vi "Periodic Tasks.vi"(11 "error in (no error)":errorcluster) -> ()   [LabVIEW 2012]
doc: "This VI runs in parallel to other tasks. It can contain as many user-defined periodic loops as you need. These can carry out PID or other sorts of timed response."
uses:
  <vilib>/Rock Robotics/WPI/DriverStation/DriverStationLCD/WPI_DriverStationLCDLCDLine.ctl
  <vilib>/Rock Robotics/SystemInterfaces/Utilities/FPGA_UtilitiesLED Source.ctl
  <vilib>/Rock Robotics/SystemInterfaces/Utilities/FPGA_UtilitiesLED State.ctl
  Robot Global Data.vi
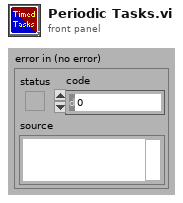
[diagram p1: front panel]
types:
  T1 = typedef "FPGA_UtilitiesLED State.ctl" = enum16{"Off", "On", "Toggle"}
  T2 = typedef "FPGA_UtilitiesLED Source.ctl" = enum16{"User LED", "FPGA LED"}
  T3 = typedef "WPI_DriverStationLCDLCDLine.ctl" = enum16{"Main - Line 1", "User - Line 2", "User - Line 3", "User - Line 4", "User - Line 5", "User - Line 6"}
  T4 = cluster{"Case":dbl, "VisionTrack":bool, "ShootEnableWheels":bool, "Shoot":bool, "ManualExtend":dbl, "ManualRotate":dbl, "YCoord":dbl, "FlipUp":bool, "RotDeadband":dbl, "ExtDeadband":dbl, "ExtPOT":dbl, "RotPOT":dbl, "WheelFSpd":dbl, "WheelBSpd":dbl, "ServoPositions":cluster{"FlipperLeftUp":dbl, "FlipperLeftDown":dbl, "FlipperRightUp":dbl, "FlipperRightDown":dbl, "KickerLeftBack":dbl, "KickerLeftForward":dbl, "KickerRightBack":dbl, "KickerRightForward":dbl}, "POTPositions":cluster{"Setpoint 1":dbl, "Setpoint 2":dbl, "Setpoint 3":dbl, "Setpoint 4":dbl, "RotLow":dbl, "RotHigh":dbl, "ExtLow":dbl, "ExtHigh":dbl}, "ClimberHooked":bool}
  T5 = typedef "WPI_DigitalInputDevRef.ctl" = cluster{"DevStatus":errorcluster, "DIO Channel":T6, "Digital Module":T7}
  T6 = typedef "FPGA_DIOChannel.ctl" = enum8{"DIO 1", "DIO 2", "DIO 3", "DIO 4", "DIO 5", "DIO 6", "DIO 7", "DIO 8", "DIO 9", "DIO 10", "DIO 11", "DIO 12", "DIO 13", "DIO 14", "Invalid"}
  T7 = typedef "FPGA_TypedefDigitalModule.ctl" = enum16{"Digital Module 1", "Digital Module 2"}
  T8 = typedef "WPI_AnalogChannelDevRef.ctl" = cluster{"DevStatus":errorcluster, "Analog Module":T9, "Analog Channel":T10}
  T9 = typedef "FPGA_TypedefAnalogModule.ctl" = enum16{"Analog Module 1", "Analog Module 2"}
  T10 = typedef "FPGA_AIChannel.ctl" = enum8{"AI 1", "AI 2", "AI 3", "AI 4", "AI 5", "AI 6", "AI 7", "AI 8", "Invalid"}
  T11 = cluster{"FlipperLeftUp":dbl, "FlipperLeftDown":dbl, "FlipperRightUp":dbl, "FlipperRightDown":dbl, "KickerLeftBack":dbl, "KickerLeftForward":dbl, "KickerRightBack":dbl, "KickerRightForward":dbl}
  T12 = cluster{"Setpoint 1":dbl, "Setpoint 2":dbl, "Setpoint 3":dbl, "Setpoint 4":dbl, "RotLow":dbl, "RotHigh":dbl, "ExtLow":dbl, "ExtHigh":dbl}
  T13 = typedef "WPI_RelayValue.ctl" = enum16{"Off", "On", "Forward", "Reverse"}
  T14 = cluster{"Case":dbl, "Extension":dbl, "Rotation":dbl, "WheelF":dbl, "WheelB":dbl, "Left Kicker":dbl, "Right Kicker":dbl, "Left Flipper":dbl, "Right Flipper":dbl, "Lights":T13}
  T15 = typedef "WPI_GyroDevRef.ctl" = cluster{"DevStatus":errorcluster, "Analog Module":T9, "Analog Channel":T10, "Offset":dbl, "Gain (VoltsPerDegree/Second)":dbl}
  T16 = typedef "WPI_EncoderDevRef.ctl" = cluster{"DevStatus":errorcluster, "EncoderIndex":T17, "CounterIndex":T18, "DistancePerCount":dbl, "Decoding Type":T19}
  T17 = typedef "FPGA_EncoderIdx.ctl" = enum8{"Enc 0", "Enc 1", "Enc 2", "Enc 3", "Invalid"}
  T18 = typedef "FPGA_CounterCtrSystemIndex.ctl" = enum8{"Ctr 0", "Ctr 1", "Ctr 2", "Ctr 3", "Ctr 4", "Ctr 5", "Ctr 6", "Ctr 7", "Invalid"}
  T19 = typedef "WPI_EncoderType.ctl" = enum16{"1x", "2x", "4x"}
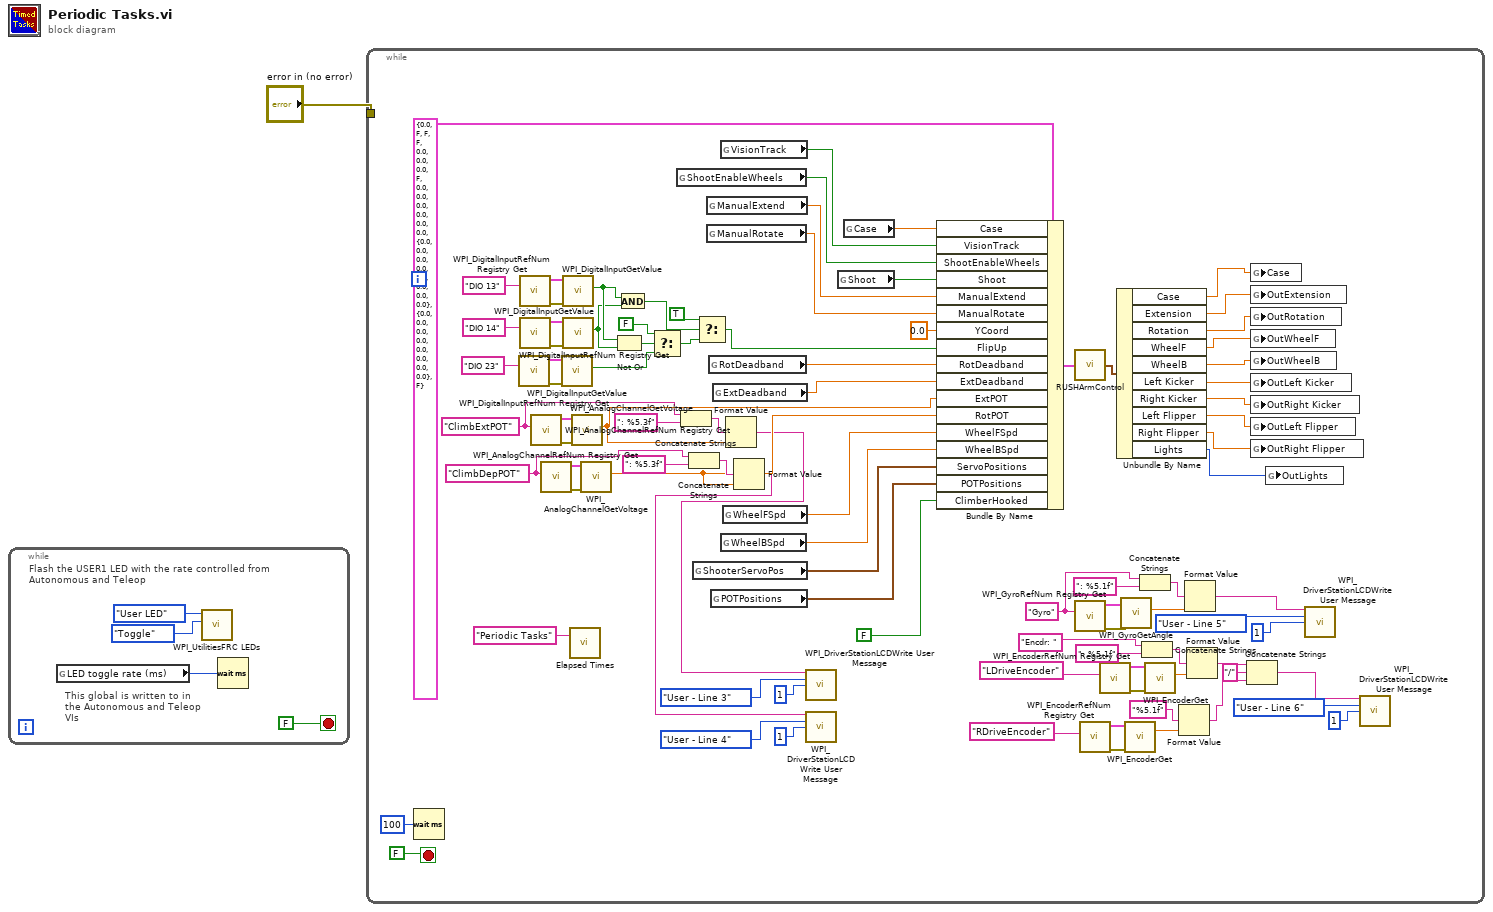
[diagram p0: block diagram]
diagram:
  n1 = while {
    stop <- FALSE stop-if-true
    # "This global is written to in the Autonomous and Teleop VIs"
    # "Flash the USER1 LED with the rate controlled from Autonomous and Teleop"
    n2 = global read "Robot Global Data.vi" "LED toggle rate (ms)"() -> (w2:u32)
    n3 = call <vilib>:"WPI_UtilitiesFRC LEDs.vi"("State"=FPGA_UtilitiesLED_State."Toggle", "LED Type"=FPGA_UtilitiesLED_Source."User LED") -> ()  [unwired: 1 in, 9 out]
    n4 = Wait (ms)(milliseconds to wait=w2) -> ()  [unwired: 1 out]
  }
  n5 = while {
    tunnel: "error in (no error)" -> [_]
    stop <- FALSE stop-if-true
    w55 = "ClimbExtPOT" ("refnum name")
    w51 = "ClimbDepPOT" ("refnum name")
    w41 = "Gyro" ("refnum name")
    n6 = Wait (ms)(milliseconds to wait=u32 100) -> ()  [unwired: 1 out]
    n7 = call <vilib>:"WPI_DigitalInputRefNum Registry Get.vi"("refnum name"="DIO 23") -> ("error out"=w24:errorcluster, "DigitalInputDevRef"=w22:T5)  [unwired: 9 in]
    n8 = call <vilib>:"WPI_DigitalInputRefNum Registry Get.vi"("refnum name"="DIO 13") -> ("error out"=w20:errorcluster, "DigitalInputDevRef"=w19:T5)  [unwired: 9 in]
    n9 = call <vilib>:"WPI_DigitalInputRefNum Registry Get.vi"("refnum name"="DIO 14") -> ("error out"=w15:errorcluster, "DigitalInputDevRef"=w16:T5)  [unwired: 9 in]
    n10 = call <vilib>:"WPI_AnalogChannelRefNum Registry Get.vi"("refnum name"=w55) -> ("error out"=w27:errorcluster, "AIDeviceRef"=w21:T8)  [unwired: 9 in]
    n11 = call <vilib>:"WPI_AnalogChannelRefNum Registry Get.vi"("refnum name"=w51) -> ("error out"=w26:errorcluster, "AIDeviceRef"=w25:T8)  [unwired: 9 in]
    n12 = call <vilib>:"WPI_DigitalInputGetValue.vi"("error in (no error)"=w24, "DigitalInputDevRef"=w22) -> ("Value"=w64:bool)  [unwired: 7 in, 2 out]
    n13 = call <vilib>:"WPI_DigitalInputGetValue.vi"("error in (no error)"=w20, "DigitalInputDevRef"=w19) -> ("Value"=w14:bool)  [unwired: 7 in, 2 out]
    n14 = call <vilib>:"WPI_DigitalInputGetValue.vi"("error in (no error)"=w15, "DigitalInputDevRef"=w16) -> ("Value"=w13:bool)  [unwired: 7 in, 2 out]
    n15 = call "Elapsed Times.vi"("Call Name"="Periodic Tasks") -> ()  [unwired: 2 in, 1 out]
    n16 = call <vilib>:"WPI_AnalogChannelGetVoltage.vi"("error in (no error)"=w27, "AIDeviceRef"=w21) -> ("Voltage"=w56:dbl)  [unwired: 7 in, 2 out]
    n17 = call <vilib>:"WPI_AnalogChannelGetVoltage.vi"("error in (no error)"=w26, "AIDeviceRef"=w25) -> ("Voltage"=w52:dbl)  [unwired: 7 in, 2 out]
    n18 = Not Or(1:w13, 2:w14) -> (0:w68:bool)
    n19 = And(x=w14, y=w13) -> (x .and. y?=w70:bool)
    n20 = Select(t=FALSE, s=w68, f=w64) -> (s? t:f=w66:bool)
    n21 = global read "Robot Global Data.vi" "ShootEnableWheels"() -> (w90:bool)
    n22 = Concatenate Strings(w55, ": %5.3f") -> (w57:string)
    n23 = Concatenate Strings(w51, ": %5.3f") -> (w54:string)
    n24 = global read "Robot Global Data.vi" "ShooterServoPos"() -> (w82:T11)
    n25 = Select(t=TRUE, s=w70, f=w66) -> (s? t:f=w65:bool)
    n26 = global read "Robot Global Data.vi" "ManualExtend"() -> (w88:dbl)
    n27 = global read "Robot Global Data.vi" "ManualRotate"() -> (w87:dbl)
    n28 = global read "Robot Global Data.vi" "RotDeadband"() -> (w86:dbl)
    n29 = global read "Robot Global Data.vi" "POTPositions"() -> (w81:T12)
    n30 = global read "Robot Global Data.vi" "ExtDeadband"() -> (w85:dbl)
    n31 = global read "Robot Global Data.vi" "VisionTrack"() -> (w91:bool)
    n32 = global read "Robot Global Data.vi" "WheelBSpd"() -> (w83:dbl)
    n33 = global read "Robot Global Data.vi" "WheelFSpd"() -> (w84:dbl)
    n34 = Format Value(format string=w57, value (0)=w56) -> (output string=w50:string)  [unwired: 1 in]
    n35 = Format Value(format string=w54, value (0)=w52) -> (output string=w49:string)  [unwired: 1 in]
    n36 = call <vilib>:"WPI_DriverStationLCDWrite User Message.vi"("line text"=w50, "line"=WPI_DriverStationLCDLCDLine."User - Line 3", "starting column"=i8 1) -> ()  [unwired: 2 in, 11 out]
    n37 = call <vilib>:"WPI_DriverStationLCDWrite User Message.vi"("line text"=w49, "line"=WPI_DriverStationLCDLCDLine."User - Line 4", "starting column"=i8 1) -> ()  [unwired: 2 in, 11 out]
    n38 = global read "Robot Global Data.vi" "Shoot"() -> (w89:bool)
    n39 = global read "Robot Global Data.vi" "Case"() -> (w92:dbl)
    n40 = Bundle By Name(cluster=T4 {"Case"=0.0, "VisionTrack"=FALSE, "ShootEnableWheels"=FALSE, "Shoot"=FALSE, "ManualExtend"=0.0, "ManualRotate"=0.0, "YCoord"=0.0, "FlipUp"=FALSE, "RotDeadband"=0.0, "ExtDeadband"=0.0, "ExtPOT"=0.0, "RotPOT"=0.0, "WheelFSpd"=0.0, "WheelBSpd"=0.0, "ServoPositions"={"FlipperLeftUp"=0.0, "FlipperLeftDown"=0.0, "FlipperRightUp"=0.0, "FlipperRightDown"=0.0, "KickerLeftBack"=0.0, "KickerLeftForward"=0.0, "KickerRightBack"=0.0, "KickerRightForward"=0.0}, "POTPositions"={"Setpoint 1"=0.0, "Setpoint 2"=0.0, "Setpoint 3"=0.0, "Setpoint 4"=0.0, "RotLow"=0.0, "RotHigh"=0.0, "ExtLow"=0.0, "ExtHigh"=0.0}, "ClimberHooked"=FALSE} ("In Cluster"), "Case"=w92, "VisionTrack"=w91, "ShootEnableWheels"=w90, "Shoot"=w89, "ManualExtend"=w88, "ManualRotate"=w87, "YCoord"=0.0, "FlipUp"=w65, "RotDeadband"=w86, "ExtDeadband"=w85, "ExtPOT"=w56, "RotPOT"=w52, "WheelFSpd"=w84, "WheelBSpd"=w83, "ServoPositions"=w82, "POTPositions"=w81, "ClimberHooked"=FALSE) -> (w94:T4)
    n41 = call "RUSHArmControl.vi"("In Cluster"=w94) -> ("Out Cluster"=w93:T14)
    n42 = call <vilib>:"WPI_GyroRefNum Registry Get.vi"("refnum name"=w41) -> ("error out"=w47:errorcluster, "GyroDevRef"=w48:T15)  [unwired: 9 in]
    n43 = call <vilib>:"WPI_EncoderRefNum Registry Get.vi"("refnum name"="RDriveEncoder") -> ("error out"=w44:errorcluster, "EncoderDevRef"=w43:T16)  [unwired: 9 in]
    n44 = call <vilib>:"WPI_EncoderRefNum Registry Get.vi"("refnum name"="LDriveEncoder") -> ("error out"=w45:errorcluster, "EncoderDevRef"=w46:T16)  [unwired: 9 in]
    n45 = Unbundle By Name(w93) -> ("Case"=w80:dbl, "Extension"=w79:dbl, "Rotation"=w78:dbl, "WheelF"=w77:dbl, "WheelB"=w76:dbl, "Left Kicker"=w75:dbl, "Right Kicker"=w74:dbl, "Left Flipper"=w73:dbl, "Right Flipper"=w72:dbl, "Lights"=w71:T13)
    n46 = call <vilib>:"WPI_GyroGetAngle.vi"("error in (no error)"=w47, "GyroDevRef"=w48) -> ("Angle"=w36:dbl)  [unwired: 6 in, 3 out]
    n47 = call <vilib>:"WPI_EncoderGet.vi"("error in (no error)"=w44, "EncoderDevRef"=w43) -> ("Distance"=w32:dbl)  [unwired: 4 in, 5 out]
    n48 = Concatenate Strings(w41, ": %5.1f") -> (w34:string)
    n49 = Concatenate Strings("Encdr: " ("string"), ": %5.1f") -> (w30:string)
    n50 = call <vilib>:"WPI_EncoderGet.vi"("error in (no error)"=w45, "EncoderDevRef"=w46) -> ("Distance"=w29:dbl)  [unwired: 4 in, 5 out]
    n51 = Format Value(format string="%5.1f", value (0)=w32) -> (output string=w9:string)  [unwired: 1 in]
    n52 = Format Value(format string=w34, value (0)=w36) -> (output string=w35:string)  [unwired: 1 in]
    n53 = Format Value(format string=w30, value (0)=w29) -> (output string=w11:string)  [unwired: 1 in]
    n54 = Concatenate Strings(w11, "/" ("string"), w9) -> (w10:string)
    n55 = global write "Robot Global Data.vi" "Case"(w80) -> ()
    n56 = global write "Robot Global Data.vi" "OutExtension"(w79) -> ()
    n57 = global write "Robot Global Data.vi" "OutRotation"(w78) -> ()
    n58 = global write "Robot Global Data.vi" "OutWheelF"(w77) -> ()
    n59 = global write "Robot Global Data.vi" "OutWheelB"(w76) -> ()
    n60 = global write "Robot Global Data.vi" "OutLeft Kicker"(w75) -> ()
    n61 = global write "Robot Global Data.vi" "OutRight Kicker"(w74) -> ()
    n62 = global write "Robot Global Data.vi" "OutLeft Flipper"(w73) -> ()
    n63 = global write "Robot Global Data.vi" "OutRight Flipper"(w72) -> ()
    n64 = global write "Robot Global Data.vi" "OutLights"(w71) -> ()
    n65 = call <vilib>:"WPI_DriverStationLCDWrite User Message.vi"("line text"=w35, "line"=WPI_DriverStationLCDLCDLine."User - Line 5", "starting column"=i8 1) -> ()  [unwired: 2 in, 11 out]
    n66 = call <vilib>:"WPI_DriverStationLCDWrite User Message.vi"("line text"=w10, "line"=WPI_DriverStationLCDLCDLine."User - Line 6", "starting column"=i8 1) -> ()  [unwired: 2 in, 11 out]
  }
